vi "Graph Color Legend.vi"(6 "Control Ref Queue":T1, 7 "Multiplot Representation In":T2, 8 "error in (no error)":errorcluster, 9 "Former Ignore States":bool, 11 "3D Plot.lvclass in":refnum<class "3D Plot.lvclass">) -> (0 "error out":errorcluster, 1 "Ignore the size change?":bool, 3 "3D Plot.lvclass out":refnum<class "3D Plot.lvclass">, 5 "Multiplot Representation Out":T2)   [LabVIEW 2020, in "3D Plot.lvclass"]
uses:
  <vilib>/Math Plots/3D Math Plots/3D Plot/3D Plot/3D Plot.lvclass
  <vilib>/Math Plots/3D Math Plots/3D Plot/3D Plot/Typedef/Multiplot Representation.ctl
  <vilib>/Math Plots/3D Math Plots/3D Plot/3D Plot/Typedef/Plot Representation.ctl
  <vilib>/Math Plots/3D Math Plots/3D Plot/3D Plot/Typedef/Range Clusters.ctl
  <vilib>/Math Plots/3D Math Plots/3D Plot/3D Plot/Typedef/Mesh Data.ctl
  <vilib>/Math Plots/3D Math Plots/3D Plot/Action String/3DMathPlot Ctrl Act Queue.ctl
  <vilib>/Math Plots/3D Math Plots/3D Plot/Action String/3DMathPlot Ctrl Act Cluster.ctl
  <vilib>/Math Plots/3D Math Plots/3D Plot/Action String/3DMathPlot State Class.ctl
  <vilib>/Math Plots/3D Math Plots/3D Plot/3D Plot/3D Plot.lvclass/3D Plot.ctl
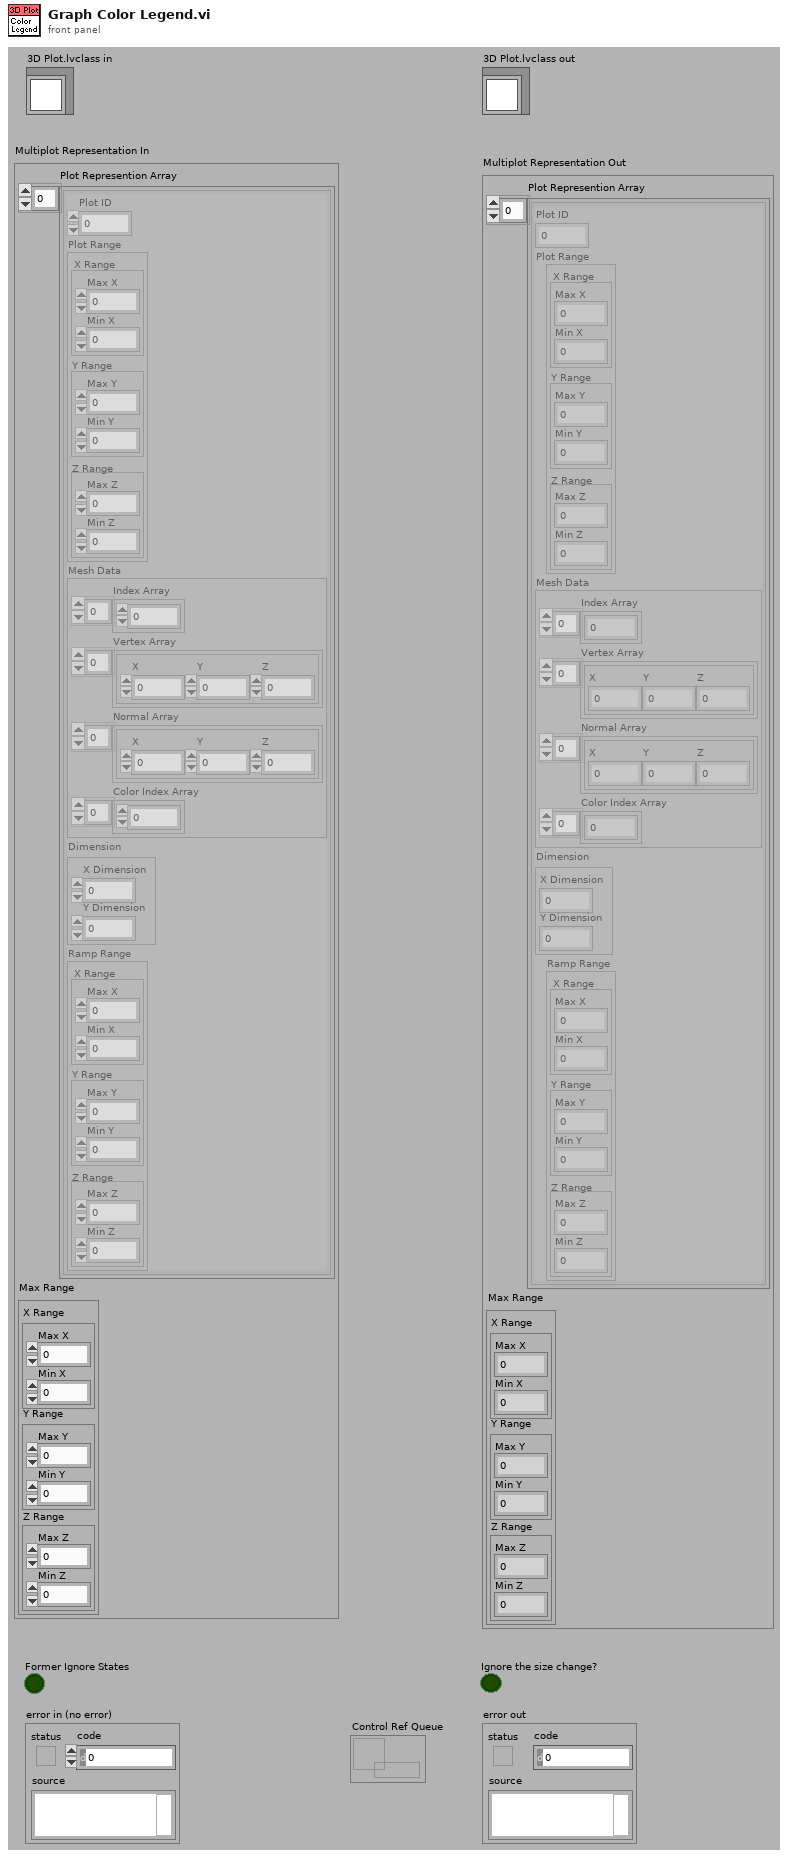
[diagram p1: front panel]
types:
  T1 = typedef "3DMathPlot Ctrl Act Queue.ctl" = refnum<queue>
  T2 = typedef "3D Plot.lvclass/Multiplot Representation.ctl" = cluster{"Plot Represention Array":T3[], "Max Range":T4}
  T3 = typedef "3D Plot.lvclass/Plot Representation.ctl" = cluster{"Plot ID":i32, "Plot Range":T4, "Mesh Data":T5, "Dimension":cluster{"X Dimension":i32, "Y Dimension":i32}, "Ramp Range":T4}
  T4 = typedef "3D Plot.lvclass/Range Clusters.ctl" = cluster{"X Range":cluster{"Max X":sgl, "Min X":sgl}, "Y Range":cluster{"Max Y":sgl, "Min Y":sgl}, "Z Range":cluster{"Max Z":sgl, "Min Z":sgl}}
  T5 = typedef "3D Plot.lvclass/Mesh Data.ctl" = cluster{"Index Array":u32[], "Vertex Array":cluster{"X":sgl, "Y":sgl, "Z":sgl}[], "Normal Array":cluster{"X":sgl, "Y":sgl, "Z":sgl}[], "Color Index Array":i32[]}
  T6 = typedef "3DMathPlot Ctrl Act Cluster.ctl" = cluster{"3D Picture Control":refnum<vi>, "Render Window Refnum":refnum<vi>, "XY Graph":refnum<vi>, "Intensity Graph":refnum<vi>, "Color Legend Palette":refnum<vi>, "Projection Palette":refnum<vi>, "XControl  Ref":refnum<vi>, "Facade Ref":refnum<vi>, "Export Image Ref":refnum<vi>, "Clear Data Flag":bool, "Display State Change Class":T7}
  T7 = typedef "3DMathPlot State Class.ctl" = enum16{"Update All Objects (Undo)", "Update Light Object Only", "Update Axis Object Only", "Update Plot Object Only", "Update Cursor Object Only", "Update Axis Plot Cursor Objects", "No Update"}
  T8 = typedef "3D Plot.lvclass/Color Ramp Cluster.ctl" = cluster{"Color Ramp Style":enum16{"None", "Shaded", "Color spectrum", "Grey scale", "Custom"}, "Color Ramp Array":u32[], "Color Ramp Index":i32[], "Interpolate?":bool, "Logarithm?":bool}
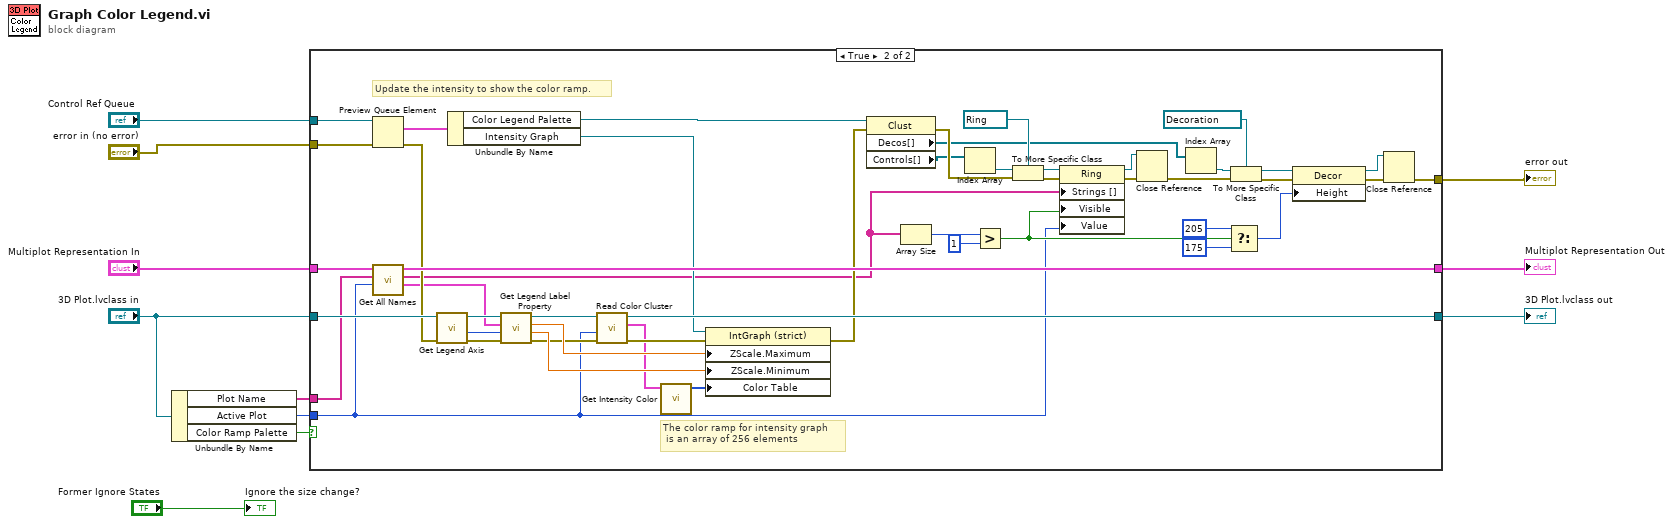
[diagram p0: block diagram]
diagram:
  n1 = Unbundle By Name("3D Plot.lvclass in") -> ("Plot Name"=w3:string[], "Active Plot"=w4:i32, "Color Ramp Palette"=w1:bool)
  n2 = case shown="True" w1 {
    tunnel: "error in (no error)" -> [w14 w62]
    tunnel: "3D Plot.lvclass in" -> [w12 w61]
    tunnel: "Multiplot Representation In" -> [w13 w60]
    tunnel: "Control Ref Queue" -> [_ w59]
    tunnel: [w12 w58] -> w7
    tunnel: [w13 w57] -> w5
    tunnel: w4 -> [_ w24]
    tunnel: w3 -> [_ w22]
    tunnel: [w14 w15] -> w2
    frame False {
    }
    frame True {
      # "The color ramp for intensity graph\n is an array of 256 elements"
      # "Update the intensity to show the color ramp."
      n3 = Preview Queue Element(queue=w59, error in (no error)=w62) -> (element=w39:T6, error out=w29:errorcluster)  [unwired: 3 out]
      n4 = call <vilib>:"Get All Names.vi"("Active Plot"=w24, "Plot Name In"=w22, "Multiplot Representation In"=w60) -> ("Plot Range"=w21:T4, "Plot Name Out"=w23:string[], "Multiplot Representation Out"=w57:T2)  [unwired: 6 in]
      n5 = call-dynamic "Get Legend Axis.vi"("error in (no error)"=w29, "3D Plot in"=w61) -> ("error out"=w30:errorcluster, "Active Axis"=w31:enum16{"X-axis", "Y-axis", "Z-axis"}, "3D Plot out"=w32:refnum<class "3D Plot.lvclass">)  [unwired: 7 out]
      n6 = Unbundle By Name(w39) -> ("Color Legend Palette"=w41:refnum<vi>, "Intensity Graph"=w40:refnum<vi>)
      n7 = call <vilib>:"Get Legend Label Property.vi"("error in (no error)"=w30, "Active Axis"=w31, "Plot Range"=w21, "3D Plot in"=w32) -> ("error out"=w33:errorcluster, "Range Min"=w34:sgl, "Range Max"=w35:sgl, "3D Plot out"=w36:refnum<class "3D Plot.lvclass">)  [unwired: 4 out]
      n8 = call-dynamic "Read Color Cluster.vi"("error in (no error)"=w33, "Active Plot"=w24, "3D Plot in"=w36) -> ("error out"=w37:errorcluster, "Color Ramp Cluster"=w28:T8, "3D Plot out"=w58:refnum<class "3D Plot.lvclass">)  [unwired: 6 out]
      n9 = call <vilib>:"Get Intensity Color.vi"("Color Ramp Cluster"=w28) -> ("Intensity Color"=w38:u32[])  [unwired: 2 in, 8 out]
      n10 = property class="IntGraph (strict)"(reference=w40, error in=w37, "ZScale.Maximum"=w35, "ZScale.Minimum"=w34, "Color Table"=w38) -> (error out=w52:errorcluster)  [unwired: 1 out]
      n11 = property class="Clust"(reference=w41, error in=w52) -> (error out=w51:errorcluster, "Decos[]"=w45:refnum<vi>[], "Controls[]"=w43:refnum<vi>[])  [unwired: 1 out]
      n12 = Array Size(array=w23) -> (size(s)=w27:i32)
      n13 = Index Array(array=w43) -> (element=w42:refnum<vi>)  [unwired: 1 in]
      n14 = Greater?(x=w27, y=1 ("x")) -> (0:w26:bool)
      n15 = To More Specific Class(target class=refnum<vi> refnum ("specific class reference"), reference=w42, error in=w51) -> (specific class reference=w53:refnum<vi>, error out=w50:errorcluster)
      n16 = property class="Ring"(reference=w53, error in=w50, "Strings []"=w23, "Visible"=w26, "Value"=w24) -> (reference out=w19:refnum<vi>, error out=w20:errorcluster)
      n17 = Close Reference(reference=w19, error in (no error)=w20) -> (error out=w18:errorcluster)
      n18 = Index Array(array=w45) -> (element=w44:refnum<vi>)  [unwired: 1 in]
      n19 = Select(t=u32 205 ("y"), s=w26, f=u32 175 ("y")) -> (s? t:f=w47:u32)
      n20 = To More Specific Class(target class=refnum<vi> refnum ("specific class reference"), reference=w44, error in=w18) -> (specific class reference=w48:refnum<vi>, error out=w46:errorcluster)
      n21 = property class="Decor"(reference=w48, error in=w46, "Height"=w47) -> (reference out=w17:refnum<vi>, error out=w16:errorcluster)
      n22 = Close Reference(reference=w17, error in (no error)=w16) -> (error out=w15:errorcluster)
    }
  }
  "error out" <- w2
  "3D Plot.lvclass out" <- w7
  "Multiplot Representation Out" <- w5
  "Ignore the size change?" <- "Former Ignore States"
